vi "Close.vi"(0 "WebSocket Connection in":refnum<k5>, 1 "timeout ms (5000)":i32=5000, 5 "Send Reason (F)":bool, 7 "Status Code":T1=1000 items=["Normal Closure"=1000, "Going Away"=1001, "Protocol Error"=1002, "Wrong Data Type"=1003, "Reserved 1004"=1004, "Reserved 1005"=1005, "Reserved 1006"=1006, "Non Consistent Data Type"=1007, "Policy Violation"=1008, "Message Too Big"=1009, "Extensions Negotiation Error"=1010, "Unexpected Condition"=1011, "Reserved 1015"=1015], 9 "Reason":string, 11 "error in (no error)":errorcluster, 12 "Mask payload?":bool) -> (4 "WebSocket Connection in":refnum<k5>, 15 "error out":errorcluster)   [LabVIEW 2017, in "LV WebSockets.lvlib"]
doc: "Sends the shutdown opcode to the TCP socket. This VI will run even if an upstream error has occurred.\n\nNote: This does not close the TCP connection as you may want to wait for the shutdown opcode to be received from the client.\nWebSockets 1.6.0.22\nSam Sharp - MediaMongrels Ltd\nCopyright (c) 2016, MediaMongrels Ltd"
uses:
  LV WebSockets.lvlib
  StatusCode.ctl
  Opcode.ctl
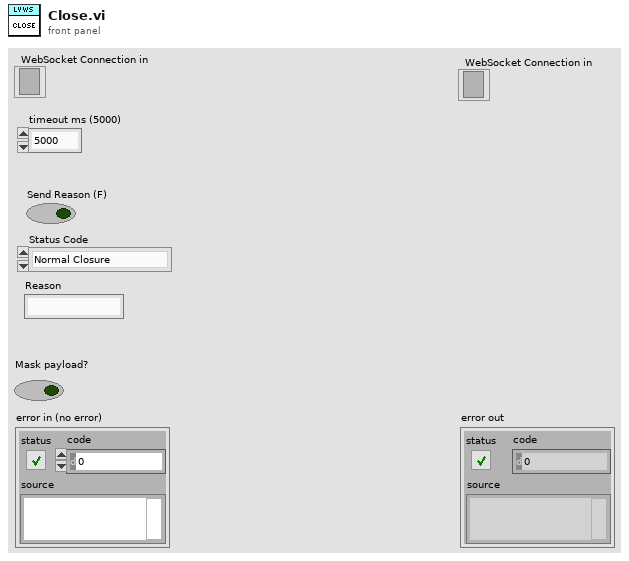
[diagram p1: front panel]
types:
  T1 = typedef "LV WebSockets.lvlib/StatusCode.ctl" = u16
  T2 = typedef "LV WebSockets.lvlib/Opcode.ctl" = enum8{"Continuation Frame", "Text Frame", "Binary Frame", "Reserved 3", "Reserved 4", "Reserved 5", "Reserved 6", "Reserved 7", "Connection Close", "Ping", "Pong", "Reserved B", "Reserved C", "Reserved D", "Reserved F"}
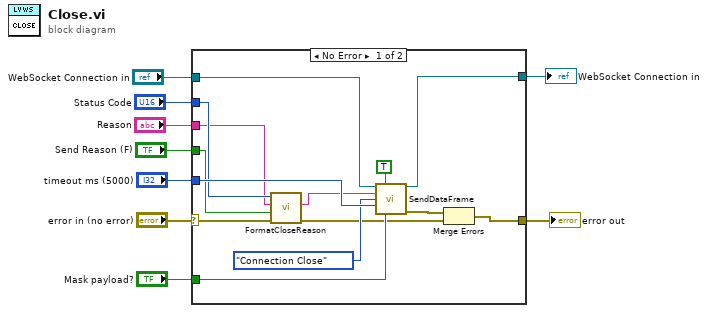
[diagram p0: block diagram]
diagram:
  n1 = case shown="No Error" "error in (no error)" {
    selector: "error in (no error)" -> [w11 w25]
    tunnel: [w23 w25] -> w8
    tunnel: [w22 w24] -> w6
    tunnel: "WebSocket Connection in" -> [w21 w24]
    tunnel: "timeout ms (5000)" -> [w20 _]
    tunnel: "Mask payload?" -> [w17 _]
    tunnel: "Status Code" -> [w15 _]
    tunnel: "Reason" -> [w14 _]
    tunnel: "Send Reason (F)" -> [w12 _]
    frame No Error {
      n2 = call "FormatCloseReason.vi"("error in (no error)"=w11, "Send Reason (F)"=w12, "Reason"=w14, "Status Code"=w15) -> ("error out"=w10:errorcluster, "Application Data"=w13:string)  [unwired: 5 in]
      n3 = call "SendDataFrame.vi"("WebSocket Connection in"=w21, "Final Frame Bit  (F)"=TRUE ("FIN Bit (F)"), "Data"=w13, "Opcode"=Opcode."Connection Close", "timeout ms (5000)"=w20, "Mask payload?"=w17) -> ("WebSocket Connection out"=w22:refnum<k5>, "error out"=w18:errorcluster)  [unwired: 8 in]
      n4 = Merge Errors(w18, w10) -> (w23:errorcluster)
    }
    frame Error {
    }
  }
  "WebSocket Connection in" <- w6
  "error out" <- w8
